vi "GearVision.vi"(8 "Turn":dbl, 9 "Forward":dbl, 11 "gearDegrees":dbl) -> (0 "gearVisionLeft":dbl, 1 "gearVisionRight":dbl, 2 "Kill":bool)   [LabVIEW 2016]
uses:
  <vilib>/Rock Robotics/Network Tables/NT Read Number.vi
  <vilib>/Rock Robotics/Network Tables/NT Write String.vi
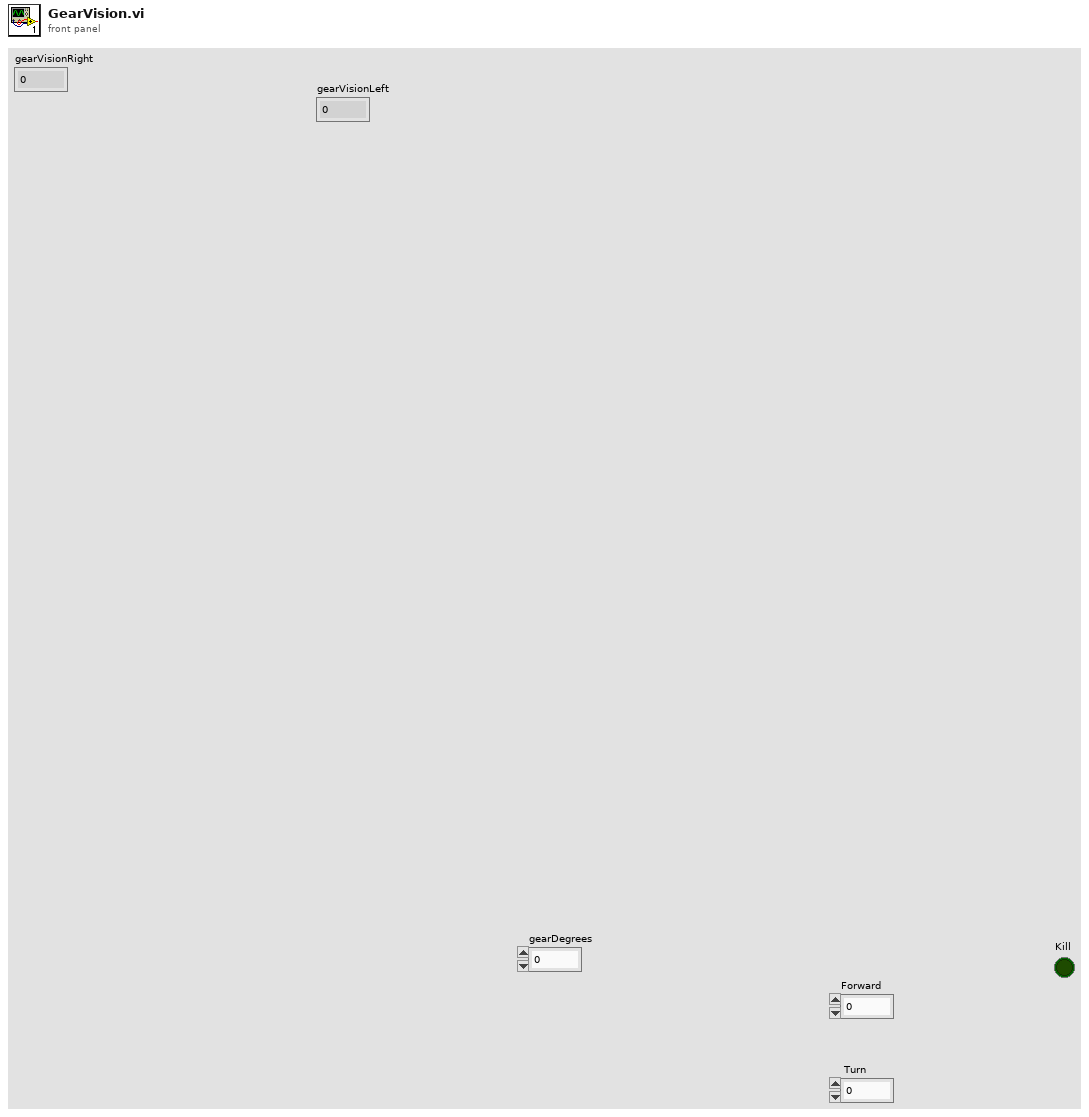
[diagram p1: front panel]
types:
  T1 = typedef "WPI_GyroDevRef.ctl" = cluster{"DevStatus":errorcluster, "Analog Channel":T2, "Offset":dbl, "Gain (VoltsPerDegree/Second)":dbl, "Gyro Type":enum16{"Analog", "XRS450"}, "Handle":i32, "SPI Bus":T3, "Device Found":bool, "Sample Rate":dbl, "Calibrate On Open":bool}
  T2 = typedef "FPGA_AIChannel.ctl" = enum8{"AI 0", "AI 1", "AI 2", "AI 3", "AI MXP 0", "AI MXP 1", "AI MXP 2", "AI MXP 3", "Invalid"}
  T3 = typedef "spi_bus.ctl" = enum16{"SPI On-Board, CS0", "SPI On-Board, CS1", "SPI On-Board, CS2", "SPI On-Board, CS3", "SPI MXP", "Invalid"}
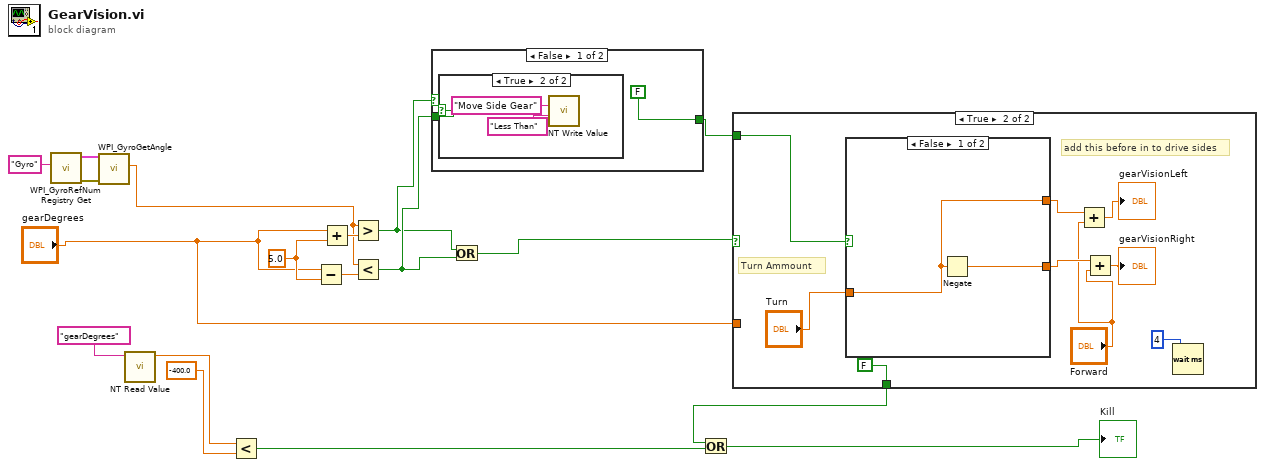
[diagram p0: block diagram]
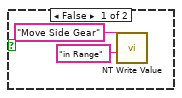
[diagram p2: hidden frame]
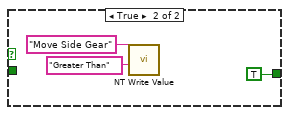
[diagram p3: hidden frame]
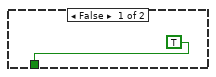
[diagram p4: hidden frame]
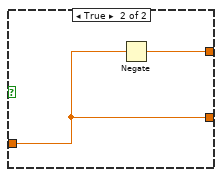
[diagram p5: hidden frame]
diagram:
  w3 = 5.0 ("y")
  n1 = call <vilib>:"WPI_GyroRefNum Registry Get.vi"("refnum name"="Gyro") -> ("error out"=w6:errorcluster, "GyroDevRef"=w5:T1)  [unwired: 9 in]
  n2 = call <vilib>:"WPI_GyroGetAngle.vi"("error in"=w6, "GyroDevRef"=w5) -> ("Angle"=w4:dbl)  [unwired: 5 in, 4 out]
  n3 = call-poly <vilib>:"NT Read Value.vi"("Name"="gearDegrees") -> ("Numeric"=w13:dbl)  [unwired: 9 in, 1 out]
  n4 = Less?(x=w13, y=-400.0) -> (x < y?=w9:bool)
  n5 = Subtract(x="gearDegrees", y=w3) -> (x-y=w12:dbl)
  n6 = Add(x="gearDegrees", y=w3) -> (x+y=w11:dbl)
  n7 = Greater?(x=w4, y=w11) -> (0:w14:bool)
  n8 = Less?(x=w4, y=w12) -> (x < y?=w15:bool)
  n9 = case shown="False" w14 {
    tunnel: w15 -> [w20 _]
    tunnel: [FALSE TRUE] -> w16
    frame False {
      n10 = case shown="True" w20 {
        frame False {
          n11 = call-poly <vilib>:"NT Write Value.vi"("String"="in Range", "Name"="Move Side Gear") -> ()  [unwired: 9 in, 1 out]
        }
        frame True {
          n12 = call-poly <vilib>:"NT Write Value.vi"("String"="Less Than", "Name"="Move Side Gear") -> ()  [unwired: 9 in, 1 out]
        }
      }
    }
    frame True {
      n13 = call-poly <vilib>:"NT Write Value.vi"("String"="Greater Than", "Name"="Move Side Gear") -> ()  [unwired: 9 in, 1 out]
    }
  }
  n14 = Or(x=w14, y=w15) -> (x .or. y?=w18:bool)
  n15 = case shown="True" w18 {
    tunnel: [TRUE FALSE] -> w17
    tunnel: "gearDegrees" -> [_ _]
    tunnel: w16 -> [_ w35]
    frame False {
    }
    frame True {
      # "Turn Ammount"
      # "add this before in to drive sides"
      n16 = case shown="False" w35 {
        tunnel: "Turn" -> [w38 w40]
        tunnel: [w38 w41] -> w31
        tunnel: [w39 w40] -> w30
        frame False {
          n17 = Negate(x=w38) -> (-x=w39:dbl)
        }
        frame True {
          n18 = Negate(x=w40) -> (-x=w41:dbl)
        }
      }
      n19 = Add(x=w31, y="Forward") -> (x+y=→"gearVisionLeft":dbl)
      n20 = Add(x=w30, y="Forward") -> (x+y=→"gearVisionRight":dbl)
      n21 = Wait (ms)(milliseconds to wait=u32 4) -> ()  [unwired: 1 out]
    }
  }
  n22 = Or(x=w17, y=w9) -> (x .or. y?=→"Kill":bool)
